vi "Network Analyzer and Frequency Tune.vi"(7 "FTUNE(ON)/NETA(OFF)":bool, 8 "Hardware Parameters In":T1={"Scan Calibration [G/V]"=0.0, "Modulation Calibration [G/V]"=0.0, "Modulation Phase [deg]"=0.0, "Modulation Frequency [Hz]"=0.0, "Attenuation [dB]"=0, "Input Channel Count"=0, "Time constant"=7, "Sensitivity"=17, "Frequency Output Voltage [V]"=0.0, "Phase Output Voltage [V]"=0.0, "Lock-in Offset Compensation"=FALSE, "RF [GHz]"=0.0, "Q Start"=0.0, "Q End"=0.0, "Balance"=0.0, "Phase Error"=0.0, "AFC Error"=0.0, "AFC"=FALSE, "Magnet Rotation"=FALSE, "Balance Scaling Factor"=1.0, "Phase Error Scaling Factor"=1.0, "AFC Error Scaling Factor"=1.0, "Frequency Counter ID"="", "Sweep Waveform"=enum."Sawtooth", "Q-Factor Scale"=0.0, " Q-Data Scale"=0.0, " Q-Data Offset"=0.0, "Magnet Rotation Slope"=0.0, "Magnet Rotation Offset"=0.0, "Phase Sweep Resolution"=0.0, "Hardware Version Number"="", "Spectrometer ID Number"=0, "Spectrometer Name"="", "Lock in Saturation"=0.0, "Balance Threshold"=0.0, "Phase Error Threshold"=0.0, "AFC Error Threshold"=0.0, "Linear Actuator Length"=0.0, "Lock-in OK?"=FALSE, "Ignore Lock-in Comm. Failure"=FALSE, "Gradient Addresses"=[], "Gradient Calibrations [G/A*mm]"=[], "Gradient Power Supplies"=[], "Lock-in Address"="", "Magnet Type"=enum."RRI", "Camera Names"=[], "Sweep Limit [Gauss]"=0.0, "Modulation Limit [Gauss]"=0.0, "Balance Threshold Exceeded?"=FALSE, "Phase Threshold Exceeded?"=FALSE, "AFC Threshold Exceeded?"=FALSE, "Consecutive Re-tune attempts"=0, "Reverse Sweep Slope [sec]"=0.0, "Reverse Sweep Offset [G]"=0.0, "AFC Field Correction [V/MHz]"=0.0, "Active Gradients (X Y Z)"=[], "SpO2 Calibration [SpO2/V]"=1.0, "Heart Rate Calibration [BPM/V]"=1.0, "Thermocouple Channel"=""} {"Sensitivity" items=["", "2 nV", "5 nV", "10 nV", "20 nV", "50 nV", "100 nV", "200 nV", "500 nV", "1 uV", "2 uV", "5 uV", "10 uV", "20 uV", "50 uV", "100 uV", "200 uV", "500 uV", "1 mV", "2 mV", "5 mV", "10 mV", "20 mV", "50 mV", "100 mV", "200 mV", "500 mV", "1 V"]; "Time constant" items=["10 us", "20 us", "40 us", "80 us", "160 us", "320 us", "640 us", "5 ms", "10 ms", "20 ms", "50 ms", "100 ms", "200 ms", "500 ms", "1 s", "2 s", "5 s", "10 s", "20 s", "50 s", "100 s", "200 s", "500 s", "1 ks", "2 ks", "5 ks", "10 ks", "20 ks", "50 ks", "100 ks"]}) -> (0 "Voltage Output":dbl=9.054, 3 "Hardware Parameters Out":T1={"Scan Calibration [G/V]"=0.0, "Modulation Calibration [G/V]"=0.0, "Modulation Phase [deg]"=0.0, "Modulation Frequency [Hz]"=0.0, "Attenuation [dB]"=0, "Input Channel Count"=0, "Time constant"=7, "Sensitivity"=17, "Frequency Output Voltage [V]"=0.0, "Phase Output Voltage [V]"=0.0, "Lock-in Offset Compensation"=FALSE, "RF [GHz]"=0.0, "Q Start"=0.0, "Q End"=0.0, "Balance"=0.0, "Phase Error"=0.0, "AFC Error"=0.0, "AFC"=FALSE, "Magnet Rotation"=FALSE, "Balance Scaling Factor"=1.0, "Phase Error Scaling Factor"=1.0, "AFC Error Scaling Factor"=1.0, "Frequency Counter ID"="", "Sweep Waveform"=enum."Sawtooth", "Q-Factor Scale"=0.0, " Q-Data Scale"=0.0, " Q-Data Offset"=0.0, "Magnet Rotation Slope"=0.0, "Magnet Rotation Offset"=0.0, "Phase Sweep Resolution"=0.0, "Hardware Version Number"="", "Spectrometer ID Number"=0, "Spectrometer Name"="", "Lock in Saturation"=0.0, "Balance Threshold"=0.0, "Phase Error Threshold"=0.0, "AFC Error Threshold"=0.0, "Linear Actuator Length"=0.0, "Lock-in OK?"=FALSE, "Ignore Lock-in Comm. Failure"=FALSE, "Gradient Addresses"=[], "Gradient Calibrations [G/A*mm]"=[], "Gradient Power Supplies"=[], "Lock-in Address"="", "Magnet Type"=enum."RRI", "Camera Names"=[], "Sweep Limit [Gauss]"=0.0, "Modulation Limit [Gauss]"=0.0, "Balance Threshold Exceeded?"=FALSE, "Phase Threshold Exceeded?"=FALSE, "AFC Threshold Exceeded?"=FALSE, "Consecutive Re-tune attempts"=0, "Reverse Sweep Slope [sec]"=0.0, "Reverse Sweep Offset [G]"=0.0, "AFC Field Correction [V/MHz]"=0.0, "Active Gradients (X Y Z)"=[], "SpO2 Calibration [SpO2/V]"=1.0, "Heart Rate Calibration [BPM/V]"=1.0, "Thermocouple Channel"=""} {"Sensitivity" items=["", "2 nV", "5 nV", "10 nV", "20 nV", "50 nV", "100 nV", "200 nV", "500 nV", "1 uV", "2 uV", "5 uV", "10 uV", "20 uV", "50 uV", "100 uV", "200 uV", "500 uV", "1 mV", "2 mV", "5 mV", "10 mV", "20 mV", "50 mV", "100 mV", "200 mV", "500 mV", "1 V"]; "Time constant" items=["10 us", "20 us", "40 us", "80 us", "160 us", "320 us", "640 us", "5 ms", "10 ms", "20 ms", "50 ms", "100 ms", "200 ms", "500 ms", "1 s", "2 s", "5 s", "10 s", "20 s", "50 s", "100 s", "200 s", "500 s", "1 ks", "2 ks", "5 ks", "10 ks", "20 ks", "50 ks", "100 ks"]})   [LabVIEW 2016]
uses:
  Types/Hardware Parameters.ctl
panel:
  in  "+16db":bool
  in  "-16db":bool
  out "Frequency Voltage Out [v]":dbl
  out "Balance Threshold Exceeded":bool
  in  "Balance Threshold":dbl
  out "railProx":bool
  out "VCenter1":dbl=9.054
  in  "secondSweep(%)":dbl=20.0
  out "secondSweep":dbl=1.0
  in  "abort":bool
  in  "Wide sweep":dbl=10.0
  out "XY Graph":cluster{"Y":dbl[], "Y":dbl[]}[](graph)
  in  "stop":bool
  out "Balance":dbl=-9.9005126953125
  # "Bridge I/O"
  # "Magnet Rotation"
  # "Field Calibration"
  # "Lock In Amplifier"
  # "Spectrometer Information"
  # "DAQ Settings"
  # "Gradient Coils and Field"
  # "X"
  # "Y"
  # "Z"
  # "Q-Measurements"
  # "Bridge I/O"
  # "Magnet Rotation"
  # "Field Calibration"
  # "Lock In Amplifier"
  # "Spectrometer Information"
  # "DAQ Settings"
  # "Gradient Coils and Field"
  # "X"
  # "Y"
  # "Z"
  # "Q-Measurements"
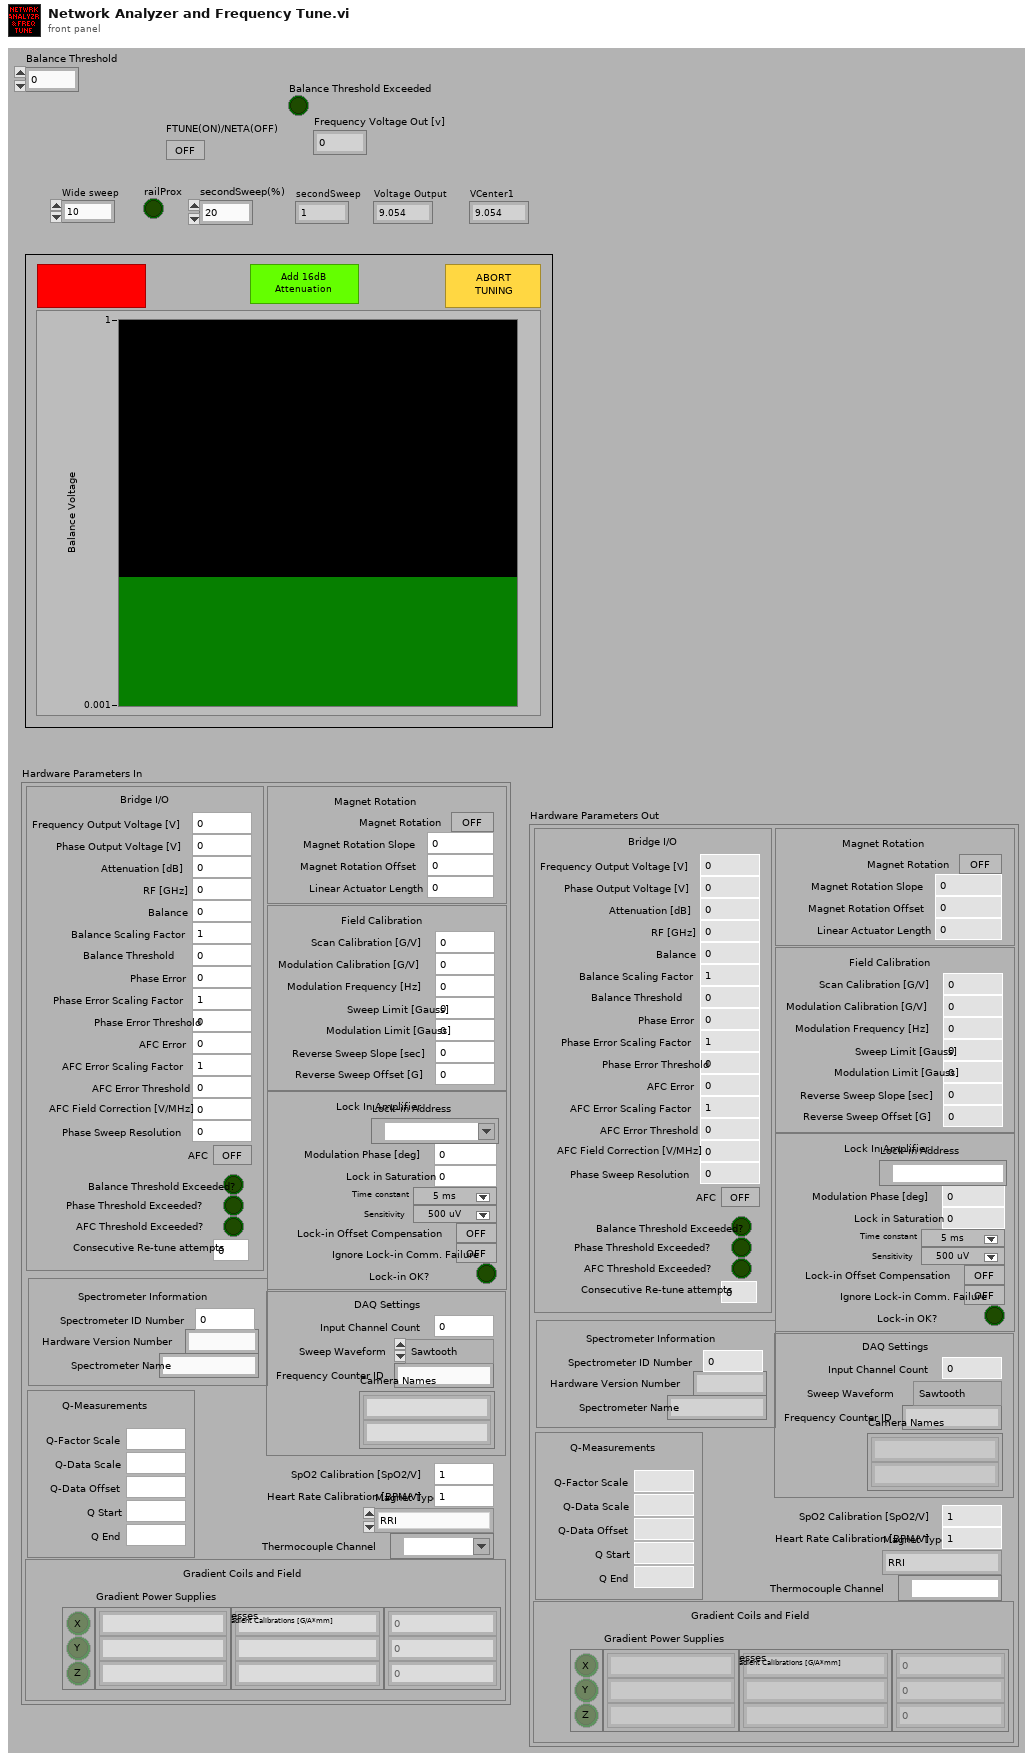
[diagram p1: front panel]
types:
  T1 = typedef "Hardware Parameters.ctl" = cluster{"Scan Calibration [G/V]":dbl, "Modulation Calibration [G/V]":dbl, "Modulation Phase [deg]":dbl, "Modulation Frequency [Hz]":dbl, "Attenuation [dB]":u16, "Input Channel Count":i32, "Time constant":u16, "Sensitivity":u16, "Frequency Output Voltage [V]":dbl, "Phase Output Voltage [V]":dbl, "Lock-in Offset Compensation":bool, "RF [GHz]":dbl, "Q Start":dbl, "Q End":dbl, "Balance":dbl, "Phase Error":dbl, "AFC Error":dbl, "AFC":bool, "Magnet Rotation":bool, "Balance Scaling Factor":dbl, "Phase Error Scaling Factor":dbl, "AFC Error Scaling Factor":dbl, "Frequency Counter ID":string, "Sweep Waveform":enum16{"Sine Wave", "Square Wave", "Sawtooth", "Triangle Wave"}, "Q-Factor Scale":dbl, " Q-Data Scale":dbl, " Q-Data Offset":dbl, "Magnet Rotation Slope":dbl, "Magnet Rotation Offset":dbl, "Phase Sweep Resolution":dbl, "Hardware Version Number":string, "Spectrometer ID Number":i32, "Spectrometer Name":string, "Lock in Saturation":dbl, "Balance Threshold":dbl, "Phase Error Threshold":dbl, "AFC Error Threshold":dbl, "Linear Actuator Length":dbl, "Lock-in OK?":bool, "Ignore Lock-in Comm. Failure":bool, "Gradient Addresses":string[], "Gradient Calibrations [G/A*mm]":dbl[], "Gradient Power Supplies":string[], "Lock-in Address":refnum<visa-resource-name>, "Magnet Type":enum16{"RRI", "BARDA", "Whole Body Permanent", "RRI Electromagnet"}, "Camera Names":string[], "Sweep Limit [Gauss]":dbl, "Modulation Limit [Gauss]":dbl, "Balance Threshold Exceeded?":bool, "Phase Threshold Exceeded?":bool, "AFC Threshold Exceeded?":bool, "Consecutive Re-tune attempts":i32, "Reverse Sweep Slope [sec]":dbl, "Reverse Sweep Offset [G]":dbl, "AFC Field Correction [V/MHz]":dbl, "Active Gradients (X Y Z)":bool[], "SpO2 Calibration [SpO2/V]":dbl, "Heart Rate Calibration [BPM/V]":dbl, "Thermocouple Channel":tag}
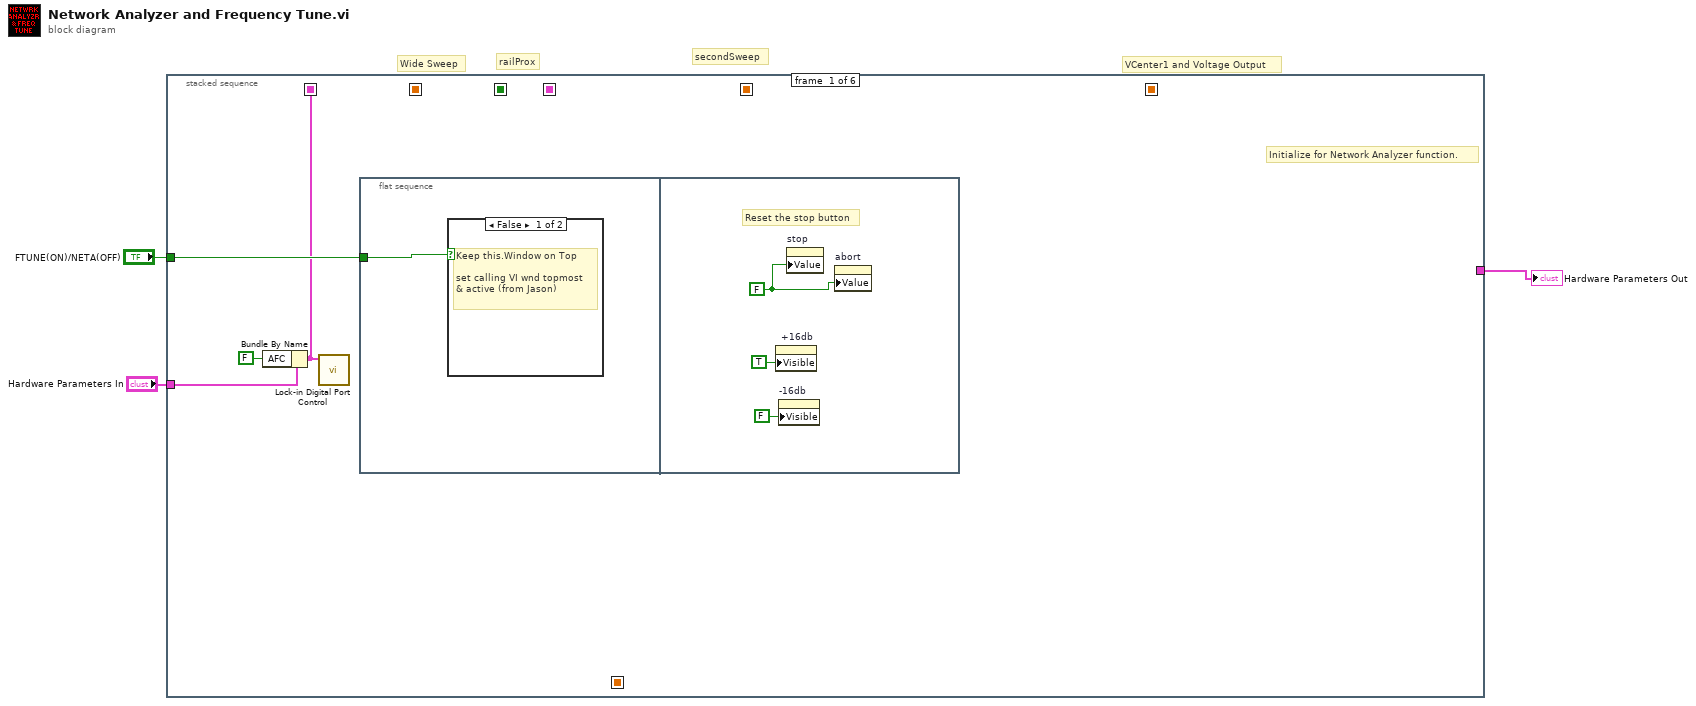
[diagram p0: block diagram]
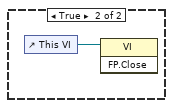
[diagram p2: hidden frame]
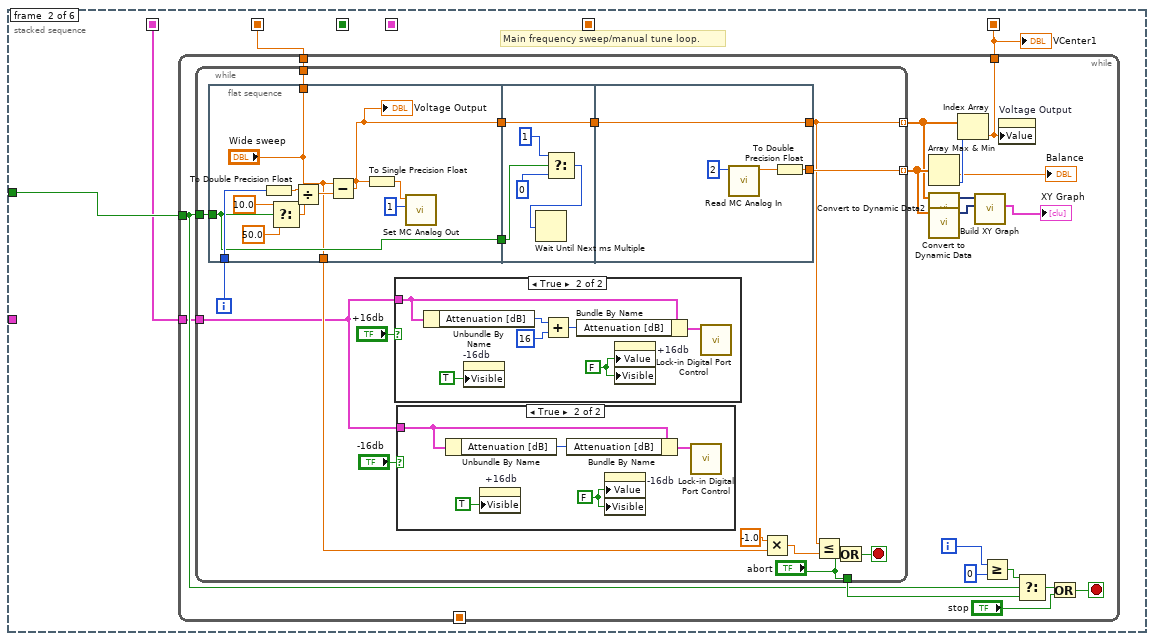
[diagram p3: hidden frame]
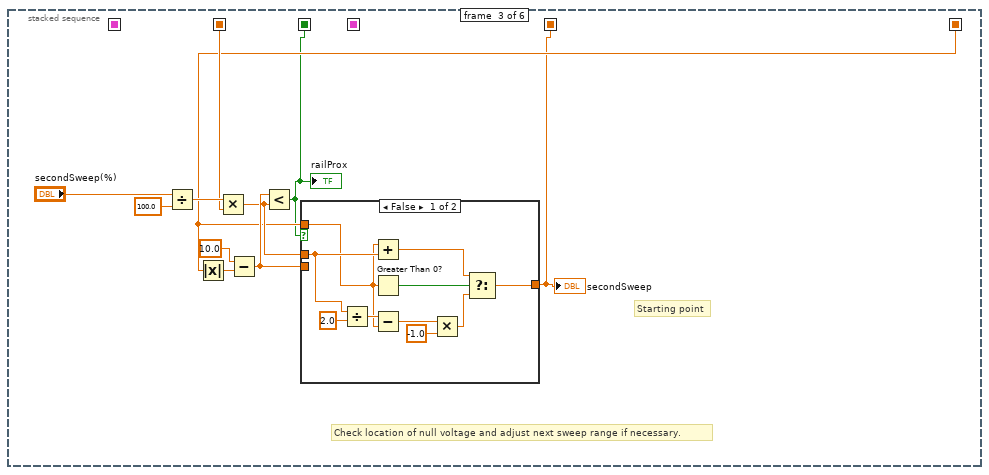
[diagram p6: hidden frame]
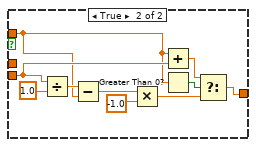
[diagram p7: hidden frame]
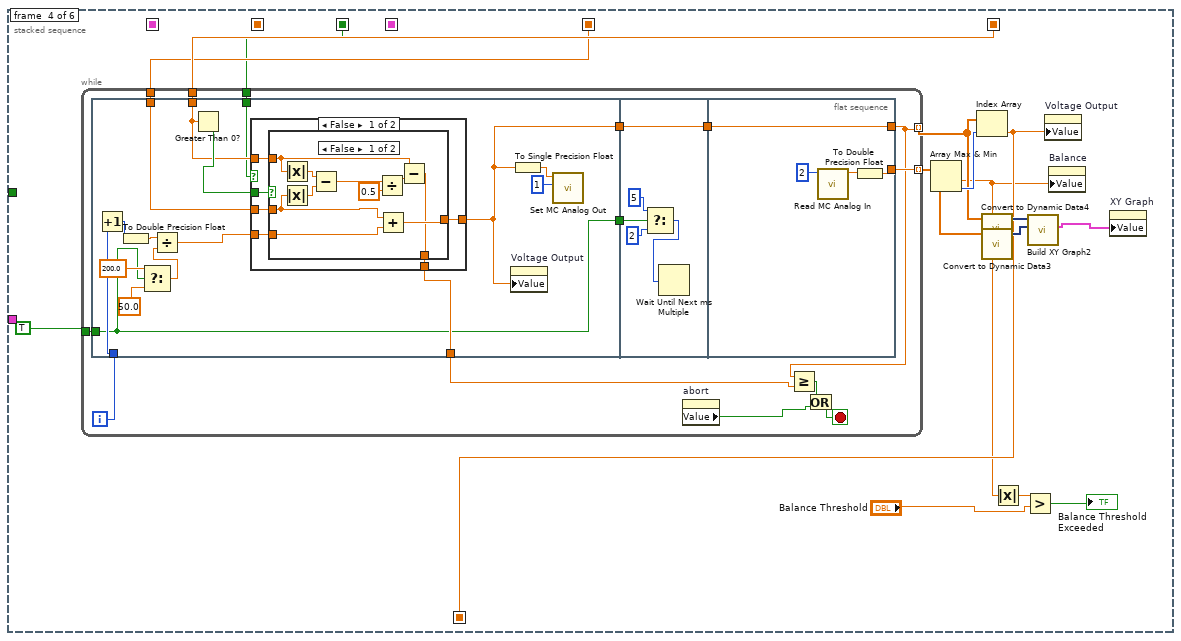
[diagram p8: hidden frame]
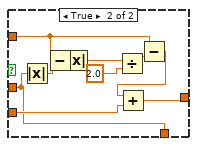
[diagram p9: hidden frame]
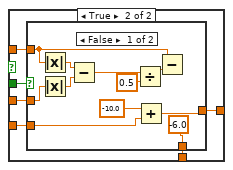
[diagram p10: hidden frame]
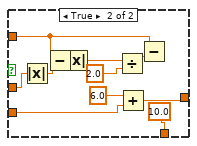
[diagram p11: hidden frame]
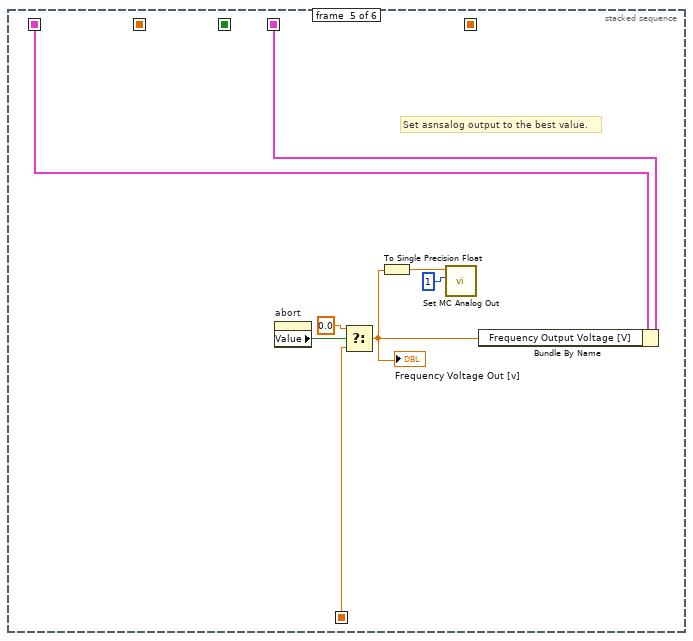
[diagram p12: hidden frame]
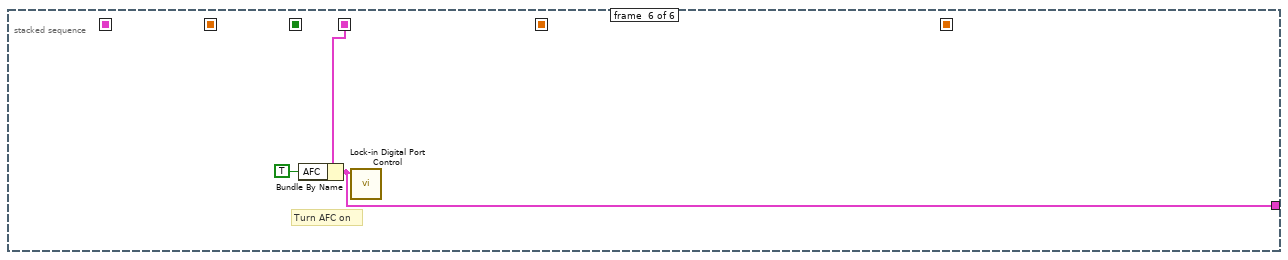
[diagram p13: hidden frame]
diagram:
  # "railProx"
  # "secondSweep"
  # "VCenter1 and Voltage Output"
  # "Wide Sweep"
  n1 = stacked-sequence {
    seq-local: [_ _ _ w118 _ _] -> [_ _ _ _ w230 _]
    seq-local: [_ w15 _ _ _ _] -> [_ _ w87 _ _ _]
    seq-local: [_ w14 _ _ _ _] -> [_ _ w86 w121 _ _]
    seq-local: [_ _ w85 _ _ _] -> [_ _ _ w120 _ _]
    seq-local: [_ _ w84 _ _ _] -> [_ _ _ w119 _ _]
    seq-local: [w4 _ _ _ _ _] -> [_ w13 _ _ w225 _]
    seq-local: [_ _ _ _ w224 _] -> [_ _ _ _ _ w232]
    tunnel: "FTUNE(ON)/NETA(OFF)" -> [w7 w16 _ _ _ _]
    tunnel: "Hardware Parameters In" -> [w5 _ _ _ _ _]
    tunnel: [_ _ _ _ _ w231] -> w1
    frame #0 {
      # "Initialize for Network Analyzer function."
      n2 = Bundle By Name(cluster=w5, "AFC"=FALSE) -> (w4:T1)
      n3 = call "Lock-in Digital Port Control.vi"("Hardware Parameters"=w4) -> ()  [unwired: 10 in, 1 out]
      n4 = flat-sequence {
        tunnel: w7 -> [w8]
        frame #0 {
          n5 = case shown="False" w8 {
            frame False {
              # "Keep this.Window on Top\n\nset calling VI wnd topmost\n& active (from Jason)"
            }
            frame True {
              n6 = control-ref of="This VI"() -> (w9:refnum<vi>)
              n7 = invoke class="VI" method="FP.Close"(reference=w9) -> ()  [unwired: 2 in, 3 out]
            }
          }
        }
        frame #1 {
          w12 = FALSE ("stop")
          # "Reset the stop button"
          n8 = property on="+16db" class="Bool (strict)"("Visible"=TRUE) -> ()  [unwired: 2 in, 2 out]
          n9 = property on="-16db" class="Bool (strict)"("Visible"=FALSE) -> ()  [unwired: 2 in, 2 out]
          n10 = property on="stop" class="Bool (strict)"("Value"=w12) -> ()  [unwired: 2 in, 2 out]
          n11 = property on="abort" class="Bool (strict)"("Value"=w12) -> ()  [unwired: 2 in, 2 out]
        }
      }
    }
    frame #1 {
      # "Main frequency sweep/manual tune loop."
      n12 = while {
        tunnel: w16 -> [w23]
        tunnel: [w19] -> w15
        tunnel: [w18] -> w14
        tunnel: w13 -> [w17]
        i -> [w26]
        stop <- w29 stop-if-true
        n13 = while {
          tunnel: [w50] -> w31 mode=indexing
          tunnel: [w46] -> w30 mode=indexing
          tunnel: ["abort"] -> w25
          tunnel: w23 -> [w41]
          tunnel: [w38] -> w19
          tunnel: w17 -> [w35]
          i -> [w51]
          stop <- w42 stop-if-true
          n14 = flat-sequence {
            tunnel: [w64] -> w45
            tunnel: ["Wide sweep"] -> w49
            tunnel: w51 -> [w74]
            tunnel: w41 -> [w68]
            tunnel: [w68] -> w40
            tunnel: ["Wide sweep"] -> w38
            tunnel: w45 -> [w79]
            tunnel: [w79] -> w44
            tunnel: w40 -> [w75]
            tunnel: [w82] -> w50
            tunnel: w44 -> [w83]
            tunnel: [w83] -> w46
            frame #0 {
              n15 = To Double Precision Float(number=w74) -> (double precision float=w72:dbl)
              n16 = Select(t=10.0, s=w68, f=50.0 ("y")) -> (s? t:f=w71:dbl)
              n17 = Divide(x=w72, y=w71) -> (x/y=w73:dbl)
              n18 = Subtract(x="Wide sweep", y=w73) -> (x-y=w64:dbl)
              "Voltage Output" <- w64
              n19 = To Single Precision Float(number=w64) -> (single precision float=w65:sgl)
              n20 = call "Set MC Analog Out.vi"("Channel"=1, "Output Voltage"=w65) -> ()  [unwired: 9 in, 1 out]
            }
            frame #1 {
              n21 = Select(t=u32 1, s=w75, f=u32 0 ("Inner Loop")) -> (s? t:f=w76:u32)
              n22 = Wait Until Next ms Multiple(millisecond multiple=w76) -> ()  [unwired: 1 out]
            }
            frame #2 {
              n23 = call "Read MC Analog In.vi"("channel"=2) -> ("Voltage Input"=w80:dbl)  [unwired: 9 in, 1 out]
              n24 = To Double Precision Float(number=w80) -> (double precision float=w82:dbl)
            }
          }
          n25 = case shown="True" "+16db" {
            tunnel: w35 -> [_ w62]
            frame False {
            }
            frame True {
              w57 = FALSE ("+16db")
              n26 = Unbundle By Name(w62) -> ("Attenuation [dB]"=w61:u16)
              n27 = property on="-16db" class="Bool (strict)"("Visible"=TRUE) -> ()  [unwired: 2 in, 2 out]
              n28 = Add(x=w61, y=u16 16) -> (x+y=w59:u16)
              n29 = Bundle By Name(cluster=w62, "Attenuation [dB]"=w59) -> (w63:T1)
              n30 = property on="+16db" class="Bool (strict)"("Value"=w57, "Visible"=w57) -> ()  [unwired: 2 in, 2 out]
              n31 = call "Lock-in Digital Port Control.vi"("Hardware Parameters"=w63) -> ()  [unwired: 10 in, 1 out]
            }
          }
          n32 = case shown="True" "-16db" {
            tunnel: w35 -> [_ w55]
            frame False {
            }
            frame True {
              w53 = FALSE ("-16db")
              n33 = Unbundle By Name(w55) -> ("Attenuation [dB]"=w52:u16)
              n34 = property on="+16db" class="Bool (strict)"("Visible"=TRUE) -> ()  [unwired: 2 in, 2 out]
              n35 = Bundle By Name(cluster=w55, "Attenuation [dB]"=w52) -> (w56:T1)
              n36 = property on="-16db" class="Bool (strict)"("Value"=w53, "Visible"=w53) -> ()  [unwired: 2 in, 2 out]
              n37 = call "Lock-in Digital Port Control.vi"("Hardware Parameters"=w56) -> ()  [unwired: 10 in, 1 out]
            }
          }
          n38 = Multiply(x=-1.0, y=w49) -> (x*y=w48:dbl)
          n39 = Less Or Equal?(x=w46, y=w48) -> (x <= y?=w43:bool)
          n40 = Or(x=w43, y="abort") -> (x .or. y?=w42:bool)
        }
        n41 = Array Max & Min(array=w31) -> (min value=→"Balance":dbl, min index (indices)=w32:i32)  [unwired: 2 out]
        n42 = call "Convert to Dynamic Data2"("Array"=w30) -> ("Dynamic Data Type"=w33:dynamicdata)  [unwired: 3 out]
        n43 = call "Convert to Dynamic Data"("Array"=w31) -> ("Dynamic Data Type"=w34:dynamicdata)  [unwired: 3 out]
        n44 = Index Array(array=w30, index=w32) -> (element=w18:dbl)
        n45 = call "Build XY Graph"("Y Input"=w34, "X Input"=w33) -> ("XY Graph"=→"XY Graph":cluster{"Y":dbl[], "Y":dbl[]}[])  [unwired: 3 in, 6 out]
        n46 = Greater Or Equal?(x=w26, y=0) -> (x >= y?=w27:bool)
        n47 = property on="Voltage Output" class="DigNum (strict)"("Value"=w18) -> ()  [unwired: 2 in, 2 out]
        n48 = Select(t=w27, s=w23, f=w25) -> (s? t:f=w24:bool)
        n49 = Or(x=w24, y="stop") -> (x .or. y?=w29:bool)
      }
      "VCenter1" <- w14
    }
    frame #2 {
      # "Starting point"
      # "Check location of null voltage and adjust next sweep range if necessary."
      n50 = Divide(x="secondSweep(%)", y=100.0) -> (x/y=w91:dbl)
      n51 = Absolute Value(x=w86) -> (abs(x)=w94:dbl)
      n52 = Multiply(x=w91, y=w87) -> (x*y=w89:dbl)
      n53 = Subtract(x=10.0, y=w94) -> (x-y=w92:dbl)
      n54 = Less?(x=w92, y=w89) -> (x < y?=w84:bool)
      "railProx" <- w84
      n55 = case shown="False" w84 {
        tunnel: w92 -> [_ w114]
        tunnel: [w99 w109] -> w85
        tunnel: w89 -> [w100 _]
        tunnel: w86 -> [w95 w105]
        frame False {
          n56 = Divide(x=w100, y=2.0) -> (x/y=w104:dbl)
          n57 = Add(x=w95, y=w100) -> (x+y=w102:dbl)
          n58 = Greater Than 0?(x=w95) -> (x > 0?=w101:bool)
          n59 = Subtract(x=w104, y=w95) -> (x-y=w98:dbl)
          n60 = Multiply(x=w98, y=-1.0) -> (x*y=w97:dbl)
          n61 = Select(t=w102, s=w101, f=w97) -> (s? t:f=w99:dbl)
        }
        frame True {
          n62 = Divide(x=w114, y=1.0) -> (x/y=w113:dbl)
          n63 = Subtract(x=w113, y=w105) -> (x-y=w107:dbl)
          n64 = Multiply(x=w107, y=-1.0) -> (x*y=w108:dbl)
          n65 = Add(x=w105, y=w114) -> (x+y=w111:dbl)
          n66 = Greater Than 0?(x=w105) -> (x > 0?=w110:bool)
          n67 = Select(t=w111, s=w110, f=w108) -> (s? t:f=w109:dbl)
        }
      }
      "secondSweep" <- w85
    }
    frame #3 {
      n68 = while {
        tunnel: [w142] -> w125 mode=indexing
        tunnel: [w136] -> w126 mode=indexing
        tunnel: TRUE ("FTUNE(ON)/NETA(OFF)") -> [w135]
        tunnel: w121 -> [w133]
        tunnel: w120 -> [w132]
        tunnel: w119 -> [w131]
        i -> [w143]
        stop <- w138 stop-if-true
        n69 = flat-sequence {
          tunnel: [w144] -> w140
          tunnel: w143 -> [w159]
          tunnel: [w154] -> w137
          tunnel: w135 -> [w150]
          tunnel: [w150] -> w134
          tunnel: w133 -> [w149]
          tunnel: w132 -> [w148]
          tunnel: w131 -> [w147]
          tunnel: w140 -> [w218]
          tunnel: [w218] -> w139
          tunnel: w134 -> [w215]
          tunnel: [w221] -> w142
          tunnel: w139 -> [w222]
          tunnel: [w222] -> w136
          frame #0 {
            n70 = Increment(x=w159) -> (x+1=w157:i32)
            n71 = To Double Precision Float(number=w157) -> (double precision float=w158:dbl)
            n72 = Select(t=200.0, s=w150, f=50.0 ("y")) -> (s? t:f=w151:dbl)
            n73 = Divide(x=w158, y=w151) -> (x/y=w155:dbl)
            n74 = Greater Than 0?(x=w149) -> (x > 0?=w156:bool)
            n75 = case shown="False" w147 {
              tunnel: w156 -> [w165 w191]
              tunnel: w155 -> [w164 w190]
              tunnel: w148 -> [w163 w189]
              tunnel: [w162 w188] -> w144
              tunnel: w149 -> [w161 w187]
              tunnel: [w160 w186] -> w154
              frame False {
                n76 = case shown="False" w165 {
                  tunnel: w164 -> [w175 w185]
                  tunnel: w163 -> [w170 w176]
                  tunnel: [w174 w184] -> w162
                  tunnel: w161 -> [w169 w180]
                  tunnel: [w166 w176] -> w160
                  frame False {
                    n77 = Absolute Value(x=w169) -> (abs(x)=w171:dbl)
                    n78 = Absolute Value(x=w170) -> (abs(x)=w168:dbl)
                    n79 = Subtract(x=w171, y=w168) -> (x-y=w167:dbl)
                    n80 = Divide(x=w167, y=0.5) -> (x/y=w172:dbl)
                    n81 = Add(x=w170, y=w175) -> (x+y=w174:dbl)
                    n82 = Subtract(x=w169, y=w172) -> (x-y=w166:dbl)
                  }
                  frame True {
                    n83 = Absolute Value(x=w176) -> (abs(x)=w179:dbl)
                    n84 = Subtract(x=w180, y=w179) -> (x-y=w181:dbl)
                    n85 = Absolute Value(x=w181) -> (abs(x)=w178:dbl)
                    n86 = Divide(x=w178, y=2.0) -> (x/y=w182:dbl)
                    n87 = Subtract(x=w180, y=w182) -> (x-y=w177:dbl)
                    n88 = Add(x=w177, y=w185) -> (x+y=w184:dbl)
                  }
                }
              }
              frame True {
                n89 = case shown="False" w191 {
                  tunnel: w190 -> [w202 w213]
                  tunnel: w189 -> [w197 w205]
                  tunnel: [w201 w212] -> w188
                  tunnel: w187 -> [w196 w208]
                  tunnel: [-6.0 ("secondSweep") 10.0 ("secondSweep")] -> w186
                  frame False {
                    n90 = Absolute Value(x=w196) -> (abs(x)=w198:dbl)
                    n91 = Absolute Value(x=w197) -> (abs(x)=w195:dbl)
                    n92 = Subtract(x=w198, y=w195) -> (x-y=w194:dbl)
                    n93 = Divide(x=w194, y=0.5) -> (x/y=w199:dbl)
                    n94 = Add(x=-10.0, y=w202) -> (x+y=w201:dbl)
                    n95 = Subtract(x=w196, y=w199) -> ()  [unwired: 1 out]
                  }
                  frame True {
                    n96 = Absolute Value(x=w205) -> (abs(x)=w207:dbl)
                    n97 = Subtract(x=w208, y=w207) -> (x-y=w209:dbl)
                    n98 = Absolute Value(x=w209) -> (abs(x)=w206:dbl)
                    n99 = Divide(x=w206, y=2.0) -> (x/y=w210:dbl)
                    n100 = Add(x=6.0, y=w213) -> (x+y=w212:dbl)
                    n101 = Subtract(x=w208, y=w210) -> ()  [unwired: 1 out]
                  }
                }
              }
            }
            n102 = property on="Voltage Output" class="DigNum (strict)"("Value"=w144) -> ()  [unwired: 2 in, 2 out]
            n103 = To Single Precision Float(number=w144) -> (single precision float=w146:sgl)
            n104 = call "Set MC Analog Out.vi"("Channel"=1, "Output Voltage"=w146) -> ()  [unwired: 9 in, 1 out]
          }
          frame #1 {
            n105 = Select(t=u32 5, s=w215, f=u32 2 ("millisecond multiple")) -> (s? t:f=w214:u32)
            n106 = Wait Until Next ms Multiple(millisecond multiple=w214) -> ()  [unwired: 1 out]
          }
          frame #2 {
            n107 = call "Read MC Analog In.vi"("channel"=2) -> ("Voltage Input"=w219:dbl)  [unwired: 9 in, 1 out]
            n108 = To Double Precision Float(number=w219) -> (double precision float=w221:dbl)
          }
        }
        n109 = property on="abort" class="Bool (strict)"() -> ("Value"=w130:bool)  [unwired: 2 in, 2 out]
        n110 = Greater Or Equal?(x=w136, y=w137) -> (x >= y?=w141:bool)
        n111 = Or(x=w141, y=w130) -> (x .or. y?=w138:bool)
      }
      n112 = Array Max & Min(array=w125) -> (min value=w116:dbl, min index (indices)=w129:i32)  [unwired: 2 out]
      n113 = Index Array(array=w126, index=w129) -> (element=w118:dbl)
      n114 = call "Convert to Dynamic Data4"("Array"=w126) -> ("Dynamic Data Type"=w127:dynamicdata)  [unwired: 3 out]
      n115 = call "Convert to Dynamic Data3"("Array"=w125) -> ("Dynamic Data Type"=w128:dynamicdata)  [unwired: 3 out]
      n116 = Absolute Value(x=w116) -> (abs(x)=w122:dbl)
      n117 = Greater?(x=w122, y="Balance Threshold") -> (0:→"Balance Threshold Exceeded":bool)
      n118 = call "Build XY Graph2"("Y Input"=w128, "X Input"=w127) -> ("XY Graph"=w115:cluster{"Y":dbl[], "Y":dbl[]}[])  [unwired: 3 in, 6 out]
      n119 = property on="Voltage Output" class="DigNum (strict)"("Value"=w118) -> ()  [unwired: 2 in, 2 out]
      n120 = property on="Balance" class="DigNum (strict)"("Value"=w116) -> ()  [unwired: 2 in, 2 out]
      n121 = property on="XY Graph" class="XYGraph (strict)"("Value"=w115) -> ()  [unwired: 2 in, 2 out]
    }
    frame #4 {
      # "Set asnsalog output to the best value."
      n122 = property on="abort" class="Bool (strict)"() -> ("Value"=w228:bool)  [unwired: 2 in, 2 out]
      n123 = Select(t=0.0, s=w228, f=w230) -> (s? t:f=w223:dbl)
      "Frequency Voltage Out [v]" <- w223
      n124 = To Single Precision Float(number=w223) -> (single precision float=w227:sgl)
      n125 = call "Set MC Analog Out.vi"("Channel"=1, "Output Voltage"=w227) -> ()  [unwired: 9 in, 1 out]
      n126 = Bundle By Name(cluster=w225, "Frequency Output Voltage [V]"=w223) -> (w224:T1)
    }
    frame #5 {
      # "Turn AFC on"
      n127 = Bundle By Name(cluster=w232, "AFC"=TRUE) -> (w231:T1)
      n128 = call "Lock-in Digital Port Control.vi"("Hardware Parameters"=w231) -> ()  [unwired: 10 in, 1 out]
    }
  }
  "Hardware Parameters Out" <- w1
